vi "_Bias_health_check.vi"(11 "Bias_LO_equip":T2={"Node address"=19, "CAN Interface"="CAN0", "Cartridge band"=10, "Slave Node in"={"Address"=19, "Serial Number"=[16, -54, -27, 75, 1, 8, 0, 10]}, "ObjHandle out"=17, "POL"=1, "sb"=1, "GPIB_SM (SIS S,V)"="24", "GPIB_DMM (SIS I)"="22", "GPIB_SM (MAG I) "="25", "GPIB_SG(LO)"="19", "GPIB_PW (PAMP) "="6", "GPIB_TMP1(8ch)"="12", "GPIB_TMP2(2ch)  "="13", "WCA_avg"=10, "Rsen"=10.0, "BiasModule"=1, "LOModule "=2, "WCA_LO_FREQ_SET"={"YTO Low freq. [GHz]"=14.65, "YTO High freq. [GHz]"=17.5, "Kvco"=1, "Lock Pol."=0, "SET LO FREQ"=88.77778, "Multiplier"=6.0, "YTO (HEX)"=210, "YTO ( FREQ)"=14.796153, "NULL PLL INTEGRATOR"=TRUE}, "Res for"=0} {"Res for" items=["none", "series res", "parallel res"]; "WCA_LO_FREQ_SET"."YTO ( FREQ)" min=25 max=150 step=0.0001 format="%.3f"; "WCA_LO_FREQ_SET"."Multiplier" min=3 max=6 step=3; "WCA_LO_FREQ_SET"."SET LO FREQ" min=25 max=150 step=0.0001 format="%.3f"; "WCA_LO_FREQ_SET"."Lock Pol." items=["Lower", "Upper"]; "WCA_LO_FREQ_SET"."Kvco" items=["7.5MHz/V", "15MHz/V"]; "WCA_LO_FREQ_SET"."YTO High freq. [GHz]" format="%.3f"; "WCA_LO_FREQ_SET"."YTO Low freq. [GHz]" format="%.3f"; "LOModule" items=["Manual Gunn+PAMP"=0, "PLL GUNN+PAMP"=5, "B10Lab LO"=1, "WCA LO"=2, ""=3, "YIG発信器"=4, "none"=99]; "BiasModule" items=["B10Lab Bias"=0, "WCA BiasModule"=1, "none"=99]; "Slave Node in"."Serial Number" format="%.0x"; "Slave Node in"."Address" format="%.0x"; "Cartridge band" max=10 step=1; "Node address" format="%.0x"}) -> (3 "文字列":string="\r\n\r\nBHC,2012-01-28  10:16:49,Pol,0\nBHC,Vsis,-5.09, Isis,-40.39,\nBHC,Vsis,4.91, Isis,38.07,\nBHC,Rn,127.48 \nBHC,CLNA VD=,1.50, ID=,20.09, VG=,-0.66,\nBHC,Vmag,-4.13, Imag,-0.99,\nBHC,Vmag,2.23, Imag,0.61,\nBHC,Rmag,3961.61 \nBHC,T4K,299.23, T20/100,298.20, Tmix,297.91,\nBHC,heaterC, 93.52,\n\nBHC,2012-01-28  10:16:53,Pol,1\nBHC,Vsis,-5.06, Isis,-40.22,\nBHC,Vsis,4.93, Isis,39.28,\nBHC,Rn,125.68 \nBHC,CLNA VD=,1.50, ID=,20.09, VG=,-0.72,\nBHC,Vmag,-4.15, Imag,-1.06,\nBHC,Vmag,2.59, Imag,0.74,\nBHC,Rmag,3741.09 \nBHC,T4K,-1.00, T20/100,294.06, Tmix,298.76,\nBHC,heaterC, 97.70,\n\n")   [LabVIEW 2017]
uses:
  __sub_vi/WCA_NAOJ_sub_vi/WCA_Global.vi
  <vilib>/express/express arith-compare/Formula/XNode/ExpressFormulaBlockNode.xnode
panel:
  in  "CLNA_SET":T1={"CLNA State"=1, "SET POL0 LNA1 STAGE1 DRAIN V"=0.0, "SET POL0 LNA1 STAGE1 DRAIN C"=0.0, "SET POL0 LNA1 STAGE2 DRAIN V"=0.0, "SET POL0 LNA1 STAGE2 DRAIN C"=0.0, "SET POL0 LNA1 STAGE3 DRAIN V"=0.0, "SET POL0 LNA1 STAGE3 DRAIN C"=0.0} {"SET POL0 LNA1 STAGE3 DRAIN C" min=0 max=20 step=0.01 format="%.2f"; "SET POL0 LNA1 STAGE3 DRAIN V" min=0 max=3 step=0.01 format="%.2f"; "SET POL0 LNA1 STAGE2 DRAIN C" min=0 max=20 step=0.01 format="%.2f"; "SET POL0 LNA1 STAGE2 DRAIN V" min=0 max=3 step=0.01 format="%.2f"; "SET POL0 LNA1 STAGE1 DRAIN C" min=0 max=20 step=0.01 format="%.2f"; "SET POL0 LNA1 STAGE1 DRAIN V" min=0 max=3 step=0.01 format="%.2f"; "CLNA State" items=["Disabled", "Enabled"]}
  in  "Bias HC":T3={"Vmixer1 (mV)"=-5.0, "Vmixer 2(mV)"=5.0, "CLNA VD1"=1.5, "CLNA ID1 "=20.0, "Imag1 "=-1.0, "Imag2"=1.0, "save?"=FALSE}
  out "Link済み":bool=TRUE
  # "Vd [V]"
  # "Id [mA]"
  # "Stage 1"
  # "Stage 2"
  # "Stage 3"
  # "LO freq. [GHz]"
  # "YTO LOW\n/High Freq."
  # "ZERO Intgrtr"
  # "Node Address"
  # "Serial Number"
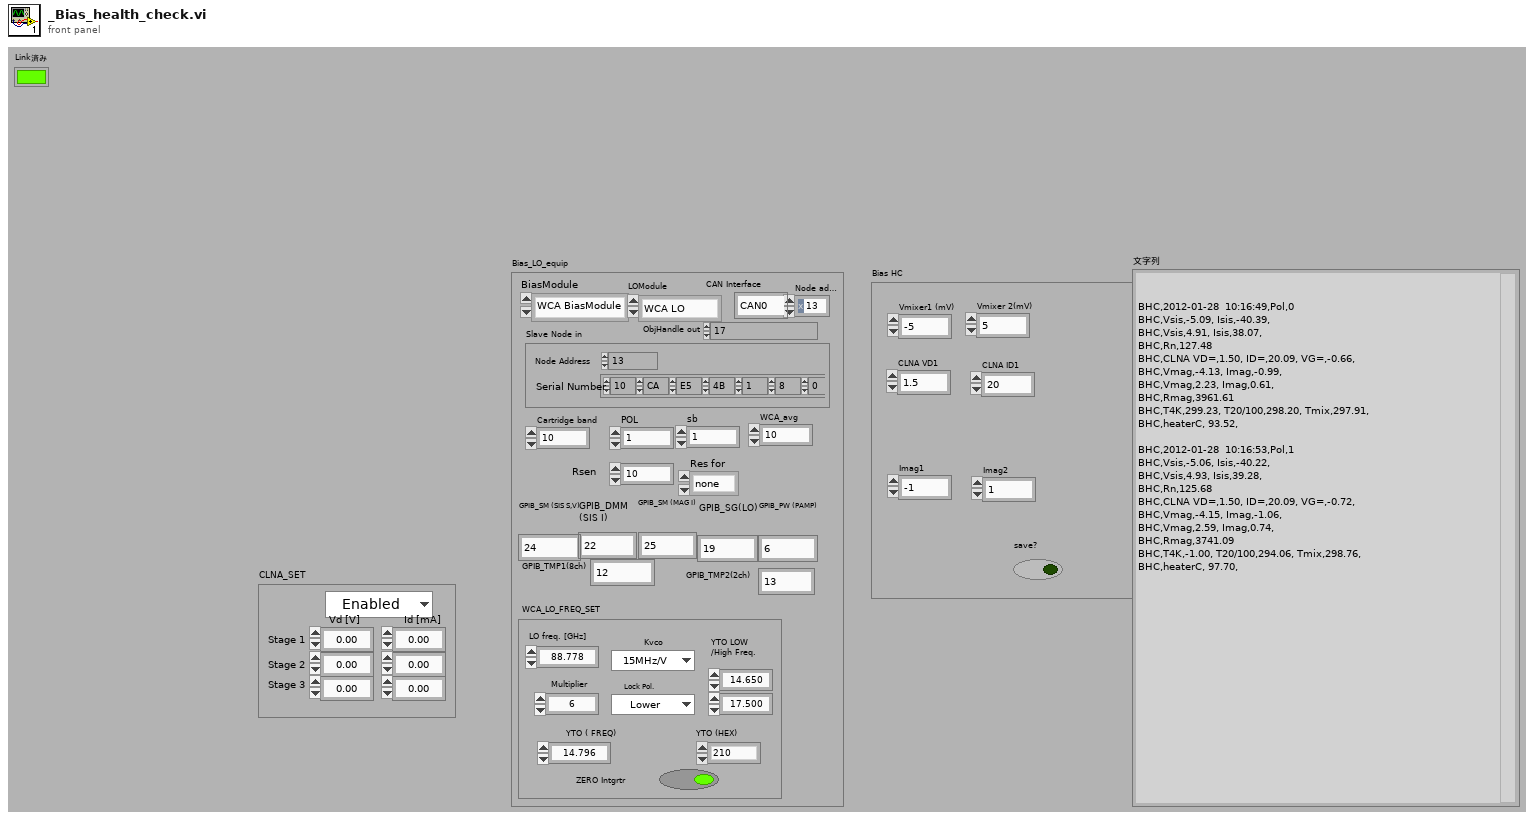
[diagram p1: front panel]
types:
  T1 = cluster{"CLNA State":u8, "SET POL0 LNA1 STAGE1 DRAIN V":sgl, "SET POL0 LNA1 STAGE1 DRAIN C":sgl, "SET POL0 LNA1 STAGE2 DRAIN V":sgl, "SET POL0 LNA1 STAGE2 DRAIN C":sgl, "SET POL0 LNA1 STAGE3 DRAIN V":sgl, "SET POL0 LNA1 STAGE3 DRAIN C":sgl}
  T2 = cluster{"Node address":u16, "CAN Interface":string, "Cartridge band":u32, "Slave Node in":cluster{"Address":i16, "Serial Number":i8[]}, "ObjHandle out":u32, "POL":u32, "sb":u32, "GPIB_SM (SIS S,V)":string, "GPIB_DMM (SIS I)":string, "GPIB_SM (MAG I) ":string, "GPIB_SG(LO)":string, "GPIB_PW (PAMP) ":string, "GPIB_TMP1(8ch)":string, "GPIB_TMP2(2ch)  ":string, "WCA_avg":i32, "Rsen":dbl, "BiasModule":u16, "LOModule ":u16, "WCA_LO_FREQ_SET":cluster{"YTO Low freq. [GHz]":sgl, "YTO High freq. [GHz]":sgl, "Kvco":u16, "Lock Pol.":u16, "SET LO FREQ":sgl, "Multiplier":sgl, "YTO (HEX)":u16, "YTO ( FREQ)":sgl, "NULL PLL INTEGRATOR":bool}, "Res for":u16}
  T3 = cluster{"Vmixer1 (mV)":dbl, "Vmixer 2(mV)":dbl, "CLNA VD1":dbl, "CLNA ID1 ":dbl, "Imag1 ":dbl, "Imag2":dbl, "save?":bool}
  T4 = cluster{"Pol0 LNA1 S1 Drain V [V]":sgl, "Pol0 LNA1 S1 Drain C [mA]":sgl, "Pol0 LNA1 S1 Gate V [V]":sgl, "Pol0 LNA1 S2 Drain V [V]":sgl, "Pol0 LNA1 S2 Drain C [mA]":sgl, "Pol0 LNA1 S2 Gate V [V]":sgl, "Pol0 LNA1 S3 Drain V [V]":sgl, "Pol0 LNA1 S3 Drain C [mA]":sgl, "Pol0 LNA1 S3 Gate V [V]":sgl, "Pol0 LNA1 State":enum16{"Disabled", "Enabled"}}
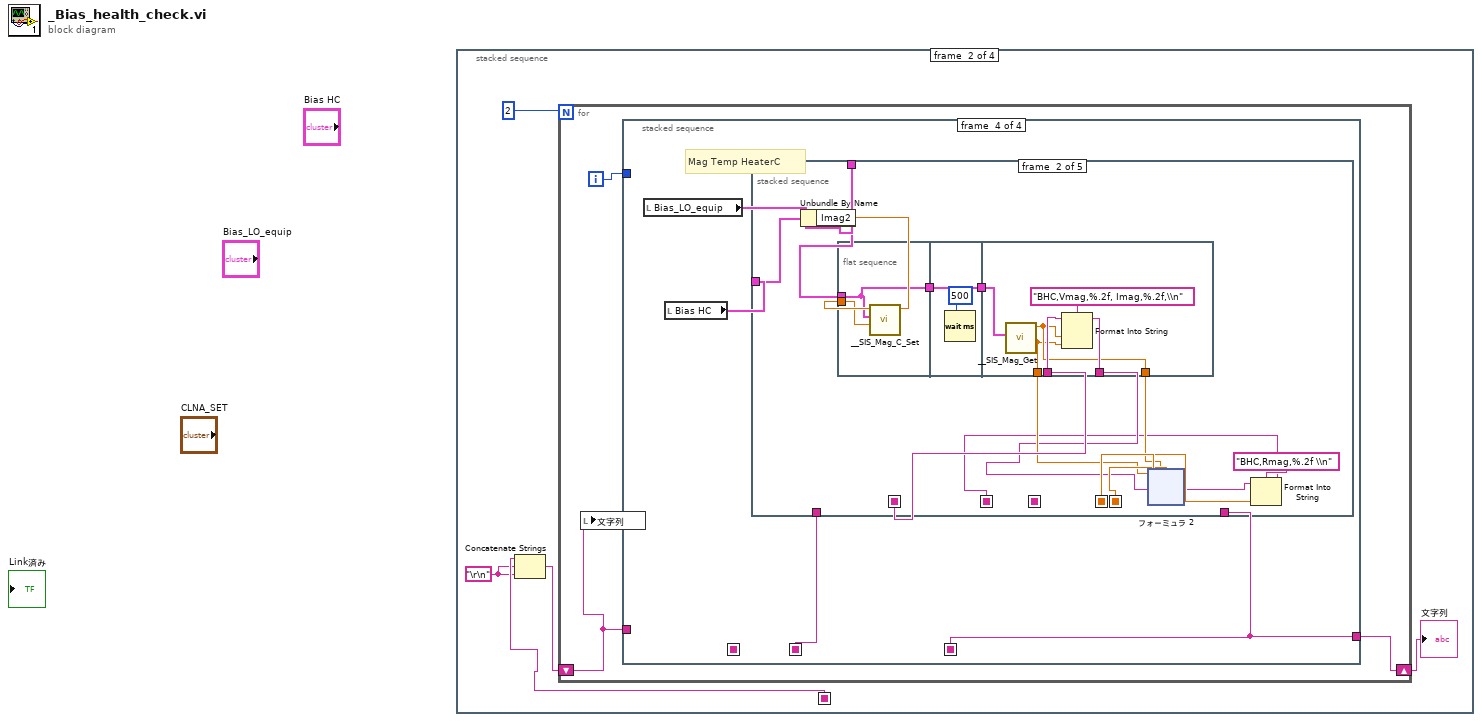
[diagram p0: block diagram]
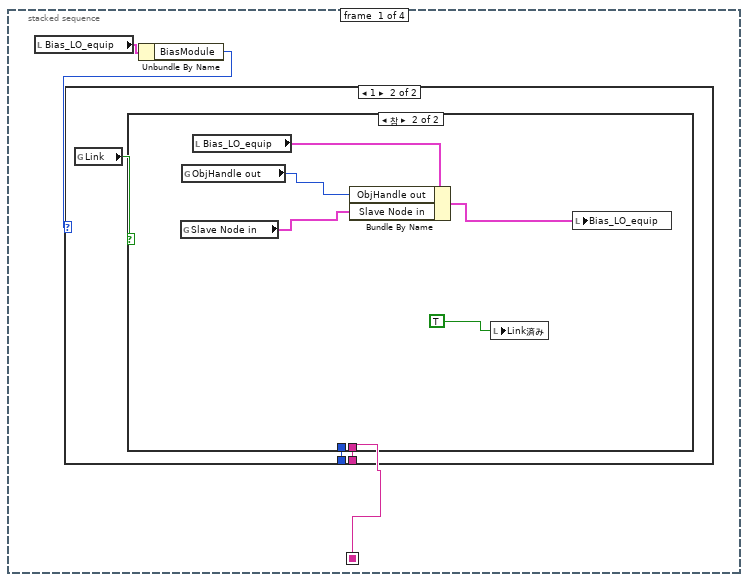
[diagram p2: hidden frame]
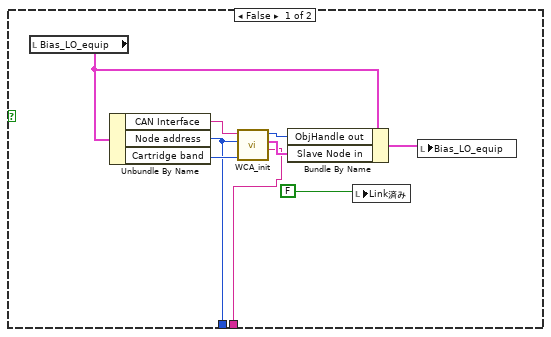
[diagram p4: hidden frame]
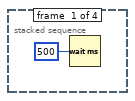
[diagram p5: hidden frame]
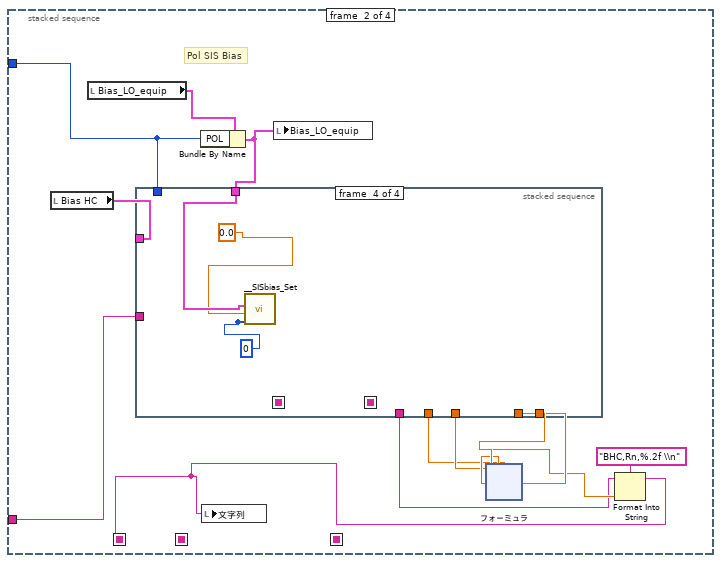
[diagram p6: hidden frame]
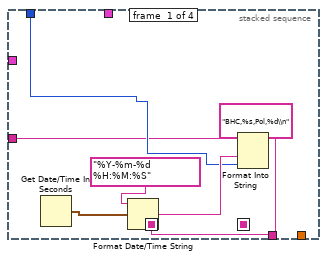
[diagram p7: hidden frame]
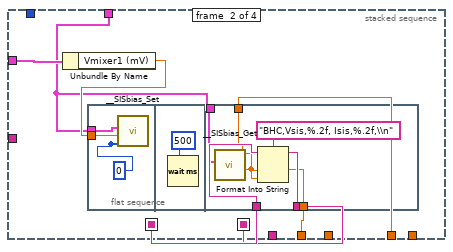
[diagram p8: hidden frame]
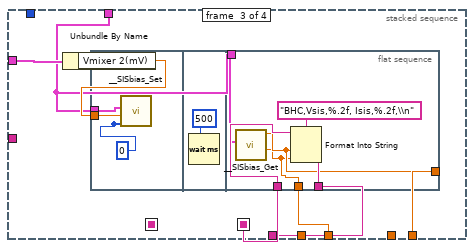
[diagram p9: hidden frame]
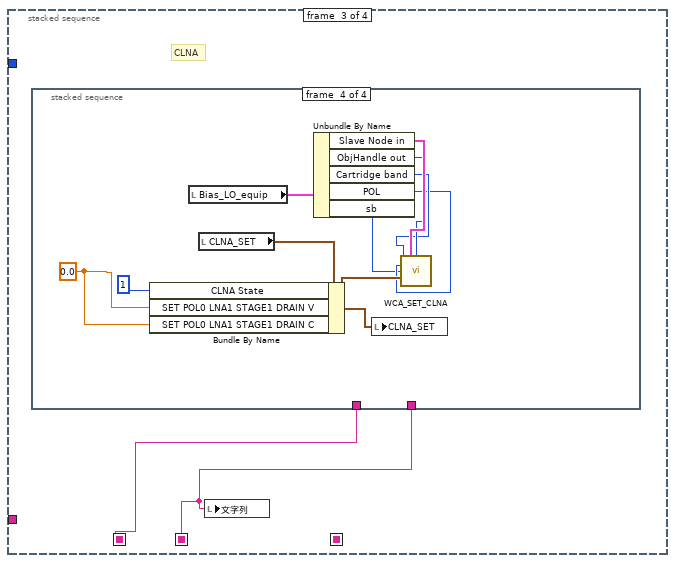
[diagram p10: hidden frame]
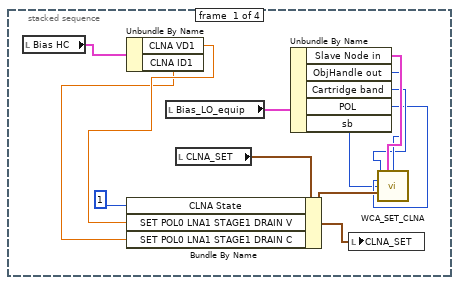
[diagram p11: hidden frame]
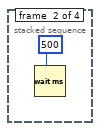
[diagram p12: hidden frame]
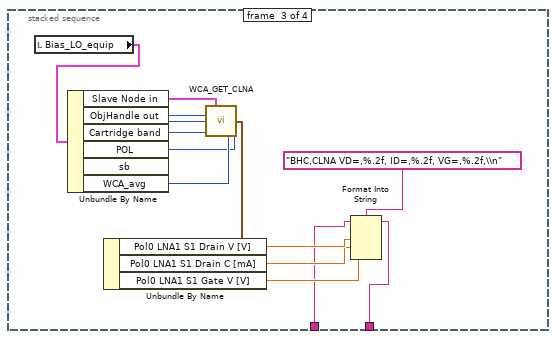
[diagram p13: hidden frame]
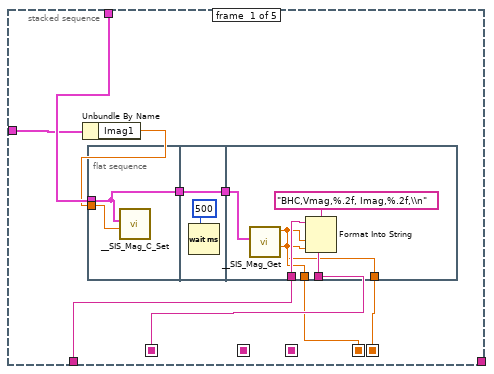
[diagram p14: hidden frame]
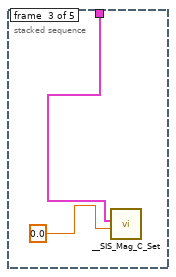
[diagram p15: hidden frame]
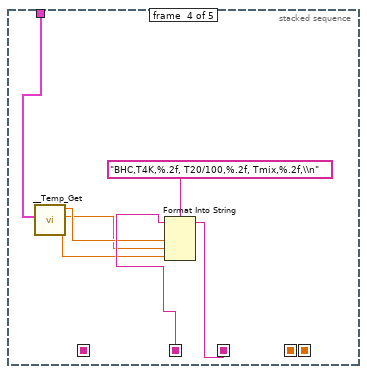
[diagram p16: hidden frame]
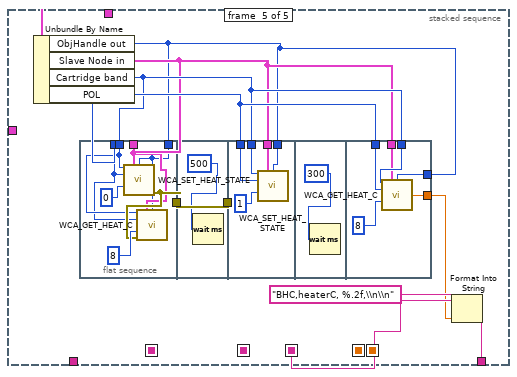
[diagram p17: hidden frame]
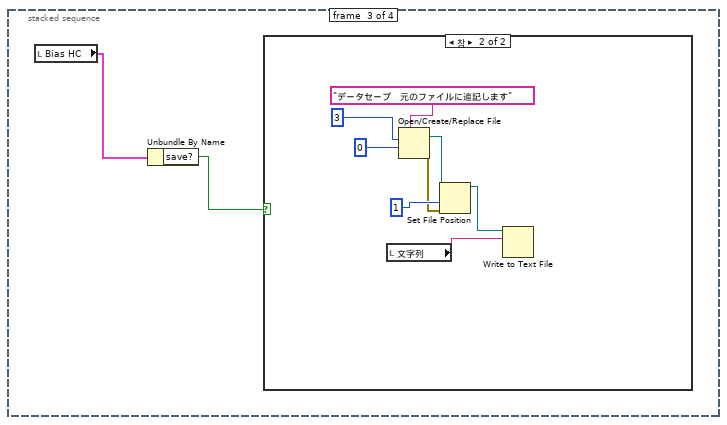
[diagram p18: hidden frame]
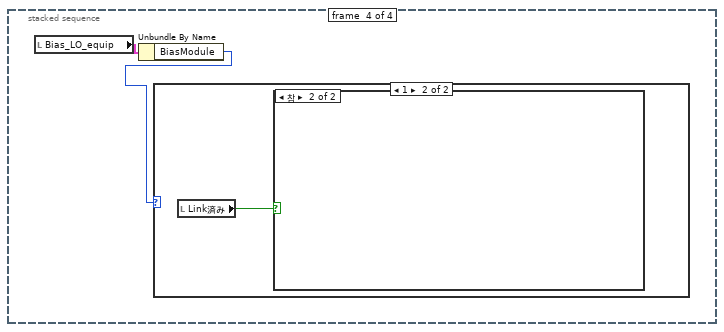
[diagram p20: hidden frame]
diagram:
  n1 = stacked-sequence {
    seq-local: [w1 _ _ _] -> [_ w23 _ _]
    frame #0 {
      n2 = local read "Bias_LO_equip"() -> (w3:T2)
      n3 = Unbundle By Name(w3) -> ("BiasModule"=w2:u16)
      n4 = case shown="1" w2 {
        tunnel: [_ w5] -> w1
        tunnel: [_ w4] -> _
        frame 0, Default {
        }
        frame 1 {
          n5 = global read "WCA_Global.vi" "Link"() -> (w6:bool)
          n6 = case shown="참" w6 {
            tunnel: [w7 _] -> w5
            tunnel: [w8 _] -> w4
            frame False {
              n7 = local read "Bias_LO_equip"() -> (w9:T2)
              n8 = Unbundle By Name(w9) -> ("CAN Interface"=w12:string, "Node address"=w8:u16, "Cartridge band"=w11:u32)
              n9 = call "WCA_init.vi"("Cartridge band"=w11, "Node address"=w8, "CAN Interface"=w12) -> ("Detected CAN Nodes."=w7:string, "Slave Node in"=w14:cluster{"Address":i16, "Serial Number":i8[]}, "ObjHandle out"=w15:u32)  [unwired: 4 in, 2 out]
              n10 = Bundle By Name(cluster=w9, "ObjHandle out"=w15, "Slave Node in"=w14) -> (w10:T2)
              n11 = local write "Link済み"(FALSE) -> ()
              n12 = local write "Bias_LO_equip"(w10) -> ()
            }
            frame True {
              n13 = global read "WCA_Global.vi" "Slave Node in"() -> (w17:cluster{"Address":i16, "Serial Number":i8[]})
              n14 = global read "WCA_Global.vi" "ObjHandle out"() -> (w18:u32)
              n15 = local read "Bias_LO_equip"() -> (w19:T2)
              n16 = Bundle By Name(cluster=w19, "ObjHandle out"=w18, "Slave Node in"=w17) -> (w20:T2)
              n17 = local write "Link済み"(TRUE) -> ()
              n18 = local write "Bias_LO_equip"(w20) -> ()
            }
          }
        }
      }
    }
    frame #1 {
      w22 = "\r\n"
      n19 = Concatenate Strings(w23, w22, w22) -> (w21:string)
      n20 = for {
        N: 2 -> [_]
        shift-right: [w27] -> w24
        shift-left: w21 -> [w26]
        i -> [w28]
        n21 = local write "文字列"(w26) -> ()
        n22 = stacked-sequence {
          seq-local: [_ w30 _ _] -> [_ _ w102 _]
          seq-local: [_ _ w101 _] -> [_ _ _ w141]
          seq-local: [_ _ _ w140] -> [_ _ _ _]
          tunnel: w28 -> [_ w39 _ _]
          tunnel: w26 -> [_ w38 _ _]
          tunnel: [_ _ _ w140] -> w27
          frame #0 {
            n23 = Wait (ms)(milliseconds to wait=500) -> ()  [unwired: 1 out]
          }
          frame #1 {
            # "Pol SIS Bias"
            n24 = local read "Bias HC"() -> (w40:T3)
            n25 = local read "Bias_LO_equip"() -> (w42:T2)
            n26 = Bundle By Name(cluster=w42, "POL"=w39) -> (w41:T2)
            n27 = stacked-sequence {
              seq-local: [w58 _ _ _] -> [_ w68 _ _]
              seq-local: [_ w67 _ _] -> [_ _ w85 _]
              tunnel: w41 -> [_ w66 w83 w100]
              tunnel: w40 -> [_ w70 w87 _]
              tunnel: w39 -> [w60 _ _ _]
              tunnel: [_ _ w84 _] -> w31
              tunnel: w38 -> [w57 _ _ _]
              tunnel: [_ w65 _ _] -> w37
              tunnel: [_ w64 _ _] -> w34
              tunnel: [_ _ w82 _] -> w36
              tunnel: [_ _ w81 _] -> w35
              frame #0 {
                n28 = Get Date/Time In Seconds() -> (seconds since 1Jan1904=w63:timestamp)
                n29 = Format Date/Time String(time format string (%c)="%Y-%m-%d  %H:%M:%S", seconds (now)=w63) -> (date/time string=w61:string)  [unwired: 1 in]
                n30 = Format Into String(format string="BHC,%s,Pol,%d\\n", initial string=w57, w61, w60) -> (resulting string=w58:string)  [unwired: 1 in, 1 out]
              }
              frame #1 {
                n31 = Unbundle By Name(w70) -> ("Vmixer1 (mV)"=w69:dbl)
                n32 = flat-sequence {
                  tunnel: w66 -> [w73]
                  tunnel: w69 -> [w72]
                  tunnel: w68 -> [w79]
                  tunnel: [w78] -> w67
                  tunnel: w66 -> [w77]
                  tunnel: [w76] -> w65
                  tunnel: [w75] -> w64
                  frame #0 {
                    w71 = 0
                    n33 = call "__SISbias_Set.vi"("SIS　Mode"=w71, "Offset"=w71, "Set_V"=w72, "Bias_LO_equip"=w73) -> ()  [unwired: 7 in, 1 out]
                  }
                  frame #1 {
                    n34 = Wait (ms)(milliseconds to wait=500) -> ()  [unwired: 1 out]
                  }
                  frame #2 {
                    n35 = call "__SISbias_Get.vi"("Bias_LO_equip"=w77) -> ("Get_I(uA)"=w75:dbl, "Get_V(mV)"=w76:dbl)  [unwired: 8 in, 1 out]
                    n36 = Format Into String(format string="BHC,Vsis,%.2f, Isis,%.2f,\\n", initial string=w79, w76, w75) -> (resulting string=w78:string)  [unwired: 1 in, 1 out]
                  }
                }
              }
              frame #2 {
                n37 = Unbundle By Name(w87) -> ("Vmixer 2(mV)"=w86:dbl)
                n38 = flat-sequence {
                  tunnel: w83 -> [w90]
                  tunnel: w86 -> [w89]
                  tunnel: w85 -> [w96]
                  tunnel: [w95] -> w84
                  tunnel: w83 -> [w94]
                  tunnel: [w93] -> w82
                  tunnel: [w92] -> w81
                  frame #0 {
                    w88 = 0
                    n39 = call "__SISbias_Set.vi"("SIS　Mode"=w88, "Offset"=w88, "Set_V"=w89, "Bias_LO_equip"=w90) -> ()  [unwired: 7 in, 1 out]
                  }
                  frame #1 {
                    n40 = Wait (ms)(milliseconds to wait=500) -> ()  [unwired: 1 out]
                  }
                  frame #2 {
                    n41 = call "__SISbias_Get.vi"("Bias_LO_equip"=w94) -> ("Get_I(uA)"=w92:dbl, "Get_V(mV)"=w93:dbl)  [unwired: 8 in, 1 out]
                    n42 = Format Into String(format string="BHC,Vsis,%.2f, Isis,%.2f,\\n", initial string=w96, w93, w92) -> (resulting string=w95:string)  [unwired: 1 in, 1 out]
                  }
                }
              }
              frame #3 {
                w99 = 0
                n43 = call "__SISbias_Set.vi"("SIS　Mode"=w99, "Offset"=w99, "Set_V"=0.0, "Bias_LO_equip"=w100) -> ()  [unwired: 7 in, 1 out]
              }
            }
            n44 = local write "Bias_LO_equip"(w41) -> ()
            n45 = xnode "フォーミュラ"("V1"=w37, "V2"=w36, "I1"=w34, "I2"=w35) -> ("結果"=w32:dbl)  [unwired: 1 in, 1 out]
            n46 = Format Into String(format string="BHC,Rn,%.2f \\n", initial string=w31, w32) -> (resulting string=w30:string)  [unwired: 1 in, 1 out]
            n47 = local write "文字列"(w30) -> ()
          }
          frame #2 {
            # "CLNA"
            n48 = stacked-sequence {
              tunnel: w102 -> [_ _ w117 _]
              tunnel: [_ _ w116 _] -> w101
              frame #0 {
                n49 = local read "Bias HC"() -> (w111:T3)
                n50 = Unbundle By Name(w111) -> ("CLNA VD1"=w104:dbl, "CLNA ID1"=w103:dbl)
                n51 = local read "Bias_LO_equip"() -> (w110:T2)
                n52 = local read "CLNA_SET"() -> (w112:T1)
                n53 = Bundle By Name(cluster=w112, "CLNA State"=1, "SET POL0 LNA1 STAGE1 DRAIN V"=w104, "SET POL0 LNA1 STAGE1 DRAIN C"=w103) -> (w113:T1)
                n54 = Unbundle By Name(w110) -> ("Slave Node in"=w109:cluster{"Address":i16, "Serial Number":i8[]}, "ObjHandle out"=w108:u32, "Cartridge band"=w107:u32, "POL"=w106:u32, "sb"=w105:u32)
                n55 = local write "CLNA_SET"(w113) -> ()
                n56 = call "WCA_SET_CLNA.vi"("Cartridge Band"=w107, "Slave Node in"=w109, "ObjHandle in"=w108, "POL"=w106, "sb"=w105, "CLNA_SET"=w113) -> ()  [unwired: 8 in, 2 out]
              }
              frame #1 {
                n57 = Wait (ms)(milliseconds to wait=500) -> ()  [unwired: 1 out]
              }
              frame #2 {
                n58 = local read "Bias_LO_equip"() -> (w123:T2)
                n59 = Unbundle By Name(w123) -> ("Slave Node in"=w129:cluster{"Address":i16, "Serial Number":i8[]}, "ObjHandle out"=w124:u32, "Cartridge band"=w125:u32, "POL"=w126:u32, "sb"=w127:u32, "WCA_avg"=w128:i32)
                n60 = call "WCA_GET_CLNA.vi"("Cartridge Band"=w125, "Slave Node in"=w129, "ObjHandle in"=w124, "POL"=w126, "sb"=w127, "avg"=w128) -> ("CLNA_monitor"=w122:T4)  [unwired: 7 in, 2 out]
                n61 = Unbundle By Name(w122) -> ("Pol0 LNA1 S1 Drain V [V]"=w120:sgl, "Pol0 LNA1 S1 Drain C [mA]"=w119:sgl, "Pol0 LNA1 S1 Gate V [V]"=w118:sgl)
                n62 = Format Into String(format string="BHC,CLNA VD=,%.2f, ID=,%.2f, VG=,%.2f,\\n", initial string=w117, w120, w119, w118) -> (resulting string=w116:string)  [unwired: 1 in, 1 out]
              }
              frame #3 {
                w130 = 0.0
                n63 = local read "Bias_LO_equip"() -> (w136:T2)
                n64 = local read "CLNA_SET"() -> (w137:T1)
                n65 = Bundle By Name(cluster=w137, "CLNA State"=1, "SET POL0 LNA1 STAGE1 DRAIN V"=w130, "SET POL0 LNA1 STAGE1 DRAIN C"=w130) -> (w138:T1)
                n66 = Unbundle By Name(w136) -> ("Slave Node in"=w135:cluster{"Address":i16, "Serial Number":i8[]}, "ObjHandle out"=w134:u32, "Cartridge band"=w133:u32, "POL"=w132:u32, "sb"=w131:u32)
                n67 = local write "CLNA_SET"(w138) -> ()
                n68 = call "WCA_SET_CLNA.vi"("Cartridge Band"=w133, "Slave Node in"=w135, "ObjHandle in"=w134, "POL"=w132, "sb"=w131, "CLNA_SET"=w138) -> ()  [unwired: 8 in, 2 out]
              }
            }
            n69 = local write "文字列"(w101) -> ()
          }
          frame #3 {
            # "Mag Temp HeaterC"
            n70 = local read "Bias_LO_equip"() -> (w142:T2)
            n71 = local read "Bias HC"() -> (w143:T3)
            n72 = stacked-sequence {
              seq-local: [w148 _ _ _ _] -> [_ w173 _ _ _]
              seq-local: [_ w163 _ _ _] -> [_ _ _ w209 _]
              seq-local: [_ _ _ w203 _] -> [_ _ _ _ w218]
              seq-local: [w145 _ _ _ _] -> [_ w169 _ _ _]
              seq-local: [w144 _ _ _ _] -> [_ w168 _ _ _]
              tunnel: w142 -> [w152 w176 w202 w207 w220]
              tunnel: w143 -> [w151 w175 _ _ _]
              tunnel: w141 -> [w149 _ _ _ _]
              tunnel: [_ _ _ _ w217] -> w140
              frame #0 {
                n73 = Unbundle By Name(w151) -> ("Imag1"=w150:dbl)
                n74 = flat-sequence {
                  tunnel: w152 -> [w153]
                  tunnel: w150 -> [w154]
                  tunnel: [w153] -> w147
                  tunnel: w147 -> [w156]
                  tunnel: [w156] -> w146
                  tunnel: [w161] -> w148
                  tunnel: w146 -> [w160]
                  tunnel: w149 -> [w159]
                  tunnel: [w158] -> w145
                  tunnel: [w157] -> w144
                  frame #0 {
                    n75 = call "__SIS_Mag_C_Set.vi"("Set_Mag_C"=w154, "Bias_LO_equip"=w153) -> ()  [unwired: 10 in]
                  }
                  frame #1 {
                    n76 = Wait (ms)(milliseconds to wait=500) -> ()  [unwired: 1 out]
                  }
                  frame #2 {
                    n77 = call "__SIS_Mag_Get.vi"("Bias_LO_equip"=w160) -> ("Get_Mag_I"=w157:dbl, "Get_Mag_V"=w158:dbl)  [unwired: 9 in]
                    n78 = Format Into String(format string="BHC,Vmag,%.2f, Imag,%.2f,\\n", initial string=w159, w158, w157) -> (resulting string=w161:string)  [unwired: 1 in, 1 out]
                  }
                }
              }
              frame #1 {
                n79 = Unbundle By Name(w175) -> ("Imag2"=w174:dbl)
                n80 = flat-sequence {
                  tunnel: w176 -> [w191]
                  tunnel: w174 -> [w192]
                  tunnel: [w191] -> w172
                  tunnel: w172 -> [w194]
                  tunnel: [w194] -> w171
                  tunnel: w171 -> [w199]
                  tunnel: w173 -> [w198]
                  tunnel: [w197] -> w164
                  tunnel: [w196] -> w167
                  tunnel: [w195] -> w166
                  frame #0 {
                    n81 = call "__SIS_Mag_C_Set.vi"("Set_Mag_C"=w192, "Bias_LO_equip"=w191) -> ()  [unwired: 10 in]
                  }
                  frame #1 {
                    n82 = Wait (ms)(milliseconds to wait=500) -> ()  [unwired: 1 out]
                  }
                  frame #2 {
                    n83 = call "__SIS_Mag_Get.vi"("Bias_LO_equip"=w199) -> ("Get_Mag_I"=w195:dbl, "Get_Mag_V"=w196:dbl)  [unwired: 9 in]
                    n84 = Format Into String(format string="BHC,Vmag,%.2f, Imag,%.2f,\\n", initial string=w198, w196, w195) -> (resulting string=w197:string)  [unwired: 1 in, 1 out]
                  }
                }
                n85 = xnode "フォーミュラ 2"("V1"=w169, "V2"=w167, "I1"=w168, "I2"=w166) -> ("結果"=w165:dbl)  [unwired: 1 in, 1 out]
                n86 = Format Into String(format string="BHC,Rmag,%.2f \\n", initial string=w164, w165) -> (resulting string=w163:string)  [unwired: 1 in, 1 out]
              }
              frame #2 {
                n87 = call "__SIS_Mag_C_Set.vi"("Set_Mag_C"=0.0, "Bias_LO_equip"=w202) -> ()  [unwired: 10 in]
              }
              frame #3 {
                n88 = call "__Temp_Get.vi"("Bias_LO_equip"=w207) -> ("MixTemp"=w204:dbl, "90/20K_temp"=w205:dbl, "4K_Temp"=w206:dbl)  [unwired: 8 in]
                n89 = Format Into String(format string="BHC,T4K,%.2f, T20/100,%.2f, Tmix,%.2f,\\n", initial string=w209, w206, w205, w204) -> (resulting string=w203:string)  [unwired: 1 in, 1 out]
              }
              frame #4 {
                n90 = Unbundle By Name(w220) -> ("ObjHandle out"=w211:u32, "Slave Node in"=w212:cluster{"Address":i16, "Serial Number":i8[]}, "Cartridge band"=w213:u32, "POL"=w214:u32)
                n91 = flat-sequence {
                  tunnel: w214 -> [w223]
                  tunnel: w213 -> [w224]
                  tunnel: w211 -> [w221]
                  tunnel: w212 -> [w222]
                  tunnel: [w225] -> w216
                  tunnel: w216 -> [w229]
                  tunnel: [w229] -> w215
                  tunnel: w215 -> [_]
                  tunnel: w213 -> [w233]
                  tunnel: w212 -> [w232]
                  tunnel: w214 -> [w231]
                  tunnel: w211 -> [w230]
                  tunnel: w214 -> [w240]
                  tunnel: w213 -> [w239]
                  tunnel: w212 -> [w238]
                  tunnel: w211 -> [w237]
                  tunnel: [w236] -> w210
                  frame #0 {
                    n92 = call "WCA_SET_HEAT_STATE.vi"("Cartridge Band"=w224, "Slave Node in"=w222, "ObjHandle in"=w221, "POL"=w223, "SET_MIX_HEAT_STATE"=0) -> ("error out"=w225:errorcluster)  [unwired: 9 in, 1 out]
                    n93 = call "WCA_GET_HEAT_C.vi"("Cartridge Band"=w224, "Slave Node in"=w222, "ObjHandle in"=w221, "POL"=w223, "avg"=8, "error in (no error)"=w225) -> ()  [unwired: 7 in, 3 out]
                  }
                  frame #1 {
                    n94 = Wait (ms)(milliseconds to wait=500) -> ()  [unwired: 1 out]
                  }
                  frame #2 {
                    n95 = call "WCA_SET_HEAT_STATE.vi"("Cartridge Band"=w233, "Slave Node in"=w232, "ObjHandle in"=w230, "POL"=w231, "SET_MIX_HEAT_STATE"=1) -> ()  [unwired: 9 in, 2 out]
                  }
                  frame #3 {
                    n96 = Wait (ms)(milliseconds to wait=300) -> ()  [unwired: 1 out]
                  }
                  frame #4 {
                    n97 = call "WCA_GET_HEAT_C.vi"("Cartridge Band"=w239, "Slave Node in"=w238, "ObjHandle in"=w237, "POL"=w240, "avg"=8) -> ("get"=w236:dbl)  [unwired: 8 in, 2 out]
                  }
                }
                n98 = Format Into String(format string="BHC,heaterC, %.2f,\\n\\n", initial string=w218, w210) -> (resulting string=w217:string)  [unwired: 1 in, 1 out]
              }
            }
          }
        }
      }
      "文字列" <- w24
    }
    frame #2 {
      n99 = local read "Bias HC"() -> (w243:T3)
      n100 = Unbundle By Name(w243) -> ("save?"=w242:bool)
      n101 = case shown="참" w242 {
        frame False {
        }
        frame True {
          n102 = local read "文字列"() -> (w251:string)
          n103 = Open/Create/Replace File(prompt="データセーブ　元のファイルに追記します", operation (0:open)=3, access (0:read/write)=0) -> (refnum out=w246:refnum<file>, error out=w249:errorcluster)  [unwired: 3 in, 1 out]
          n104 = Set File Position(refnum=w246, from (0:start)=1, error in=w249) -> (refnum out=w244:refnum<file>)  [unwired: 1 in, 1 out]
          n105 = Write to Text File(file (use dialog)=w244, text=w251) -> ()  [unwired: 2 in, 3 out]
        }
      }
    }
    frame #3 {
      n106 = local read "Bias_LO_equip"() -> (w253:T2)
      n107 = Unbundle By Name(w253) -> ("BiasModule"=w252:u16)
      n108 = case shown="1" w252 {
        frame 0, Default {
        }
        frame 1 {
          n109 = local read "Link済み"() -> (w254:bool)
          n110 = case shown="참" w254 {
            frame False {
              n111 = local read "Bias_LO_equip"() -> (w256:T2)
              n112 = Unbundle By Name(w256) -> ("ObjHandle out"=w255:u32)
              n113 = call "WCA_CAN_close.vi"("ObjHandle in"=w255) -> ()  [unwired: 14 in, 1 out]
              n114 = local write "Link済み"(FALSE) -> ()
            }
            frame True {
            }
          }
        }
      }
    }
  }
